vi "Read R Load.vi"(8 "error in (no error)":errorcluster, 11 "Heat Flow Results in":refnum<class "Heat Flow Results.lvclass">) -> (0 "error out":errorcluster, 2 "R Load":dbl, 3 "Heat Flow Results out":refnum<class "Heat Flow Results.lvclass">)   [LabVIEW 2019, in "Results.lvlib" / "Heat Flow Results.lvclass"]
uses:
  Heat Flow Results.lvclass
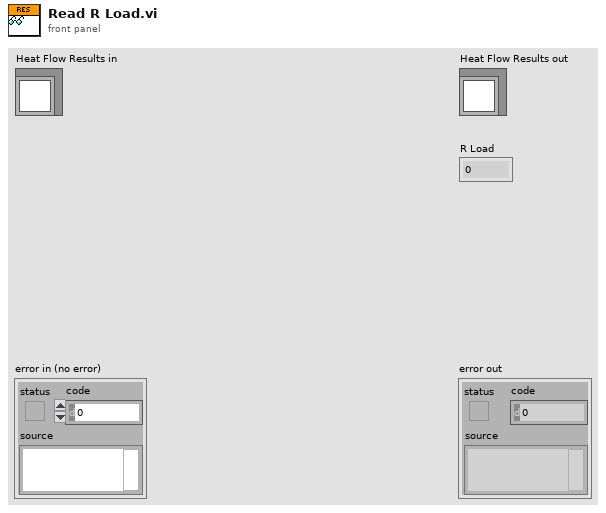
[diagram p1: front panel]
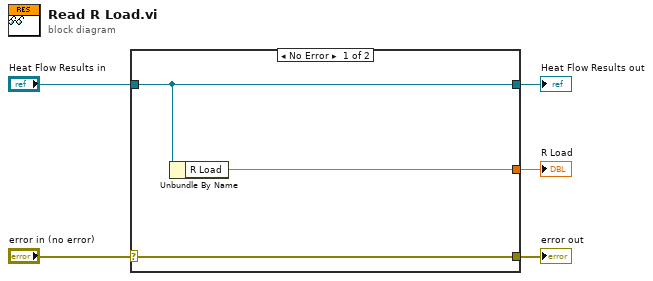
[diagram p0: block diagram]
diagram:
  n1 = case shown="No Error" "error in (no error)" {
    selector: "error in (no error)" -> [w8 w9]
    tunnel: [w8 w9] -> w4
    tunnel: [w7 w10] -> w2
    tunnel: "Heat Flow Results in" -> [w7 w10]
    tunnel: [w6 _] -> w1
    frame No Error {
      n2 = Unbundle By Name(w7) -> ("R Load"=w6:dbl)
    }
    frame Error {
    }
  }
  "error out" <- w4
  "Heat Flow Results out" <- w2
  "R Load" <- w1
